vi "TermoparRef1.vi"() -> ()   [LabVIEW 2014]
uses:
  <vilib>/Analysis/baseanly.llb/Mean (DBL).vi
  <vilib>/Analysis/NI_AALBase.lvlib
panel:
  out "Forca (Kgf)":dbl format="%#_2f"
  out "Input Voltage  Cel (V)":dbl format="%#_4f"
  in  "Numeric 4":dbl step=1.0 format="%#_3f"
  in  "Numeric 3":dbl step=1.0 format="%#_2f"
  in  "Numeric 2":dbl step=0.01 format="%#_2f"
  out "Emf(Hot Thermo B - mV)":dbl
  out "Temperature B (degC)":dbl format="%#.1f"
  out "Input Voltage Thermo B (V)":dbl format="%#_4f"
  out "Emf(Thermo B - mV)":dbl
  in  "Numeric":dbl step=0.1 format="%#_3f"
  out "Emf(Hot Thermo A - mV)":dbl
  out "Temperature A (degC)":dbl format="%#.1f"
  out "Input Voltage  Thermo A (V)":dbl format="%#_4f"
  out "Emf(Thermo A - mV)":dbl
  out "LM35 temperature (degC)":dbl format="%#_3f"
  in  "stop":bool
  out "Emf(Cold - mV)":dbl
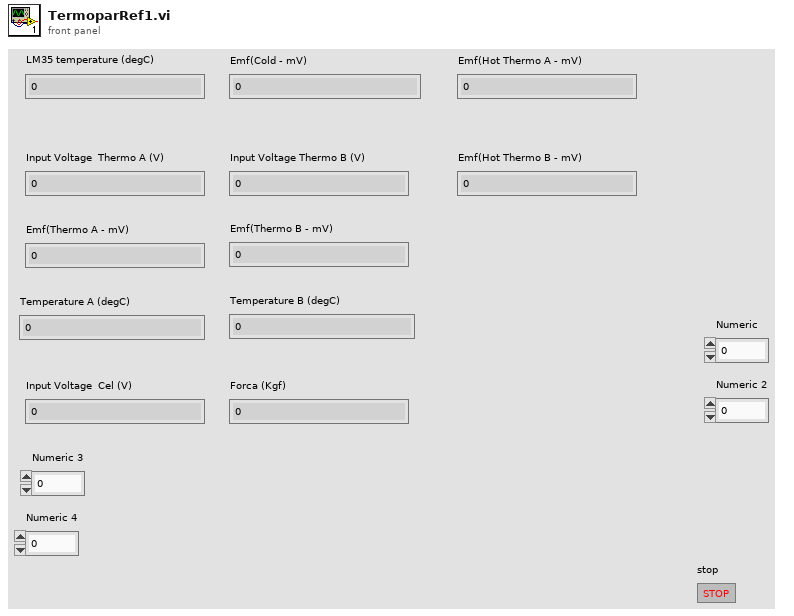
[diagram p1: front panel]
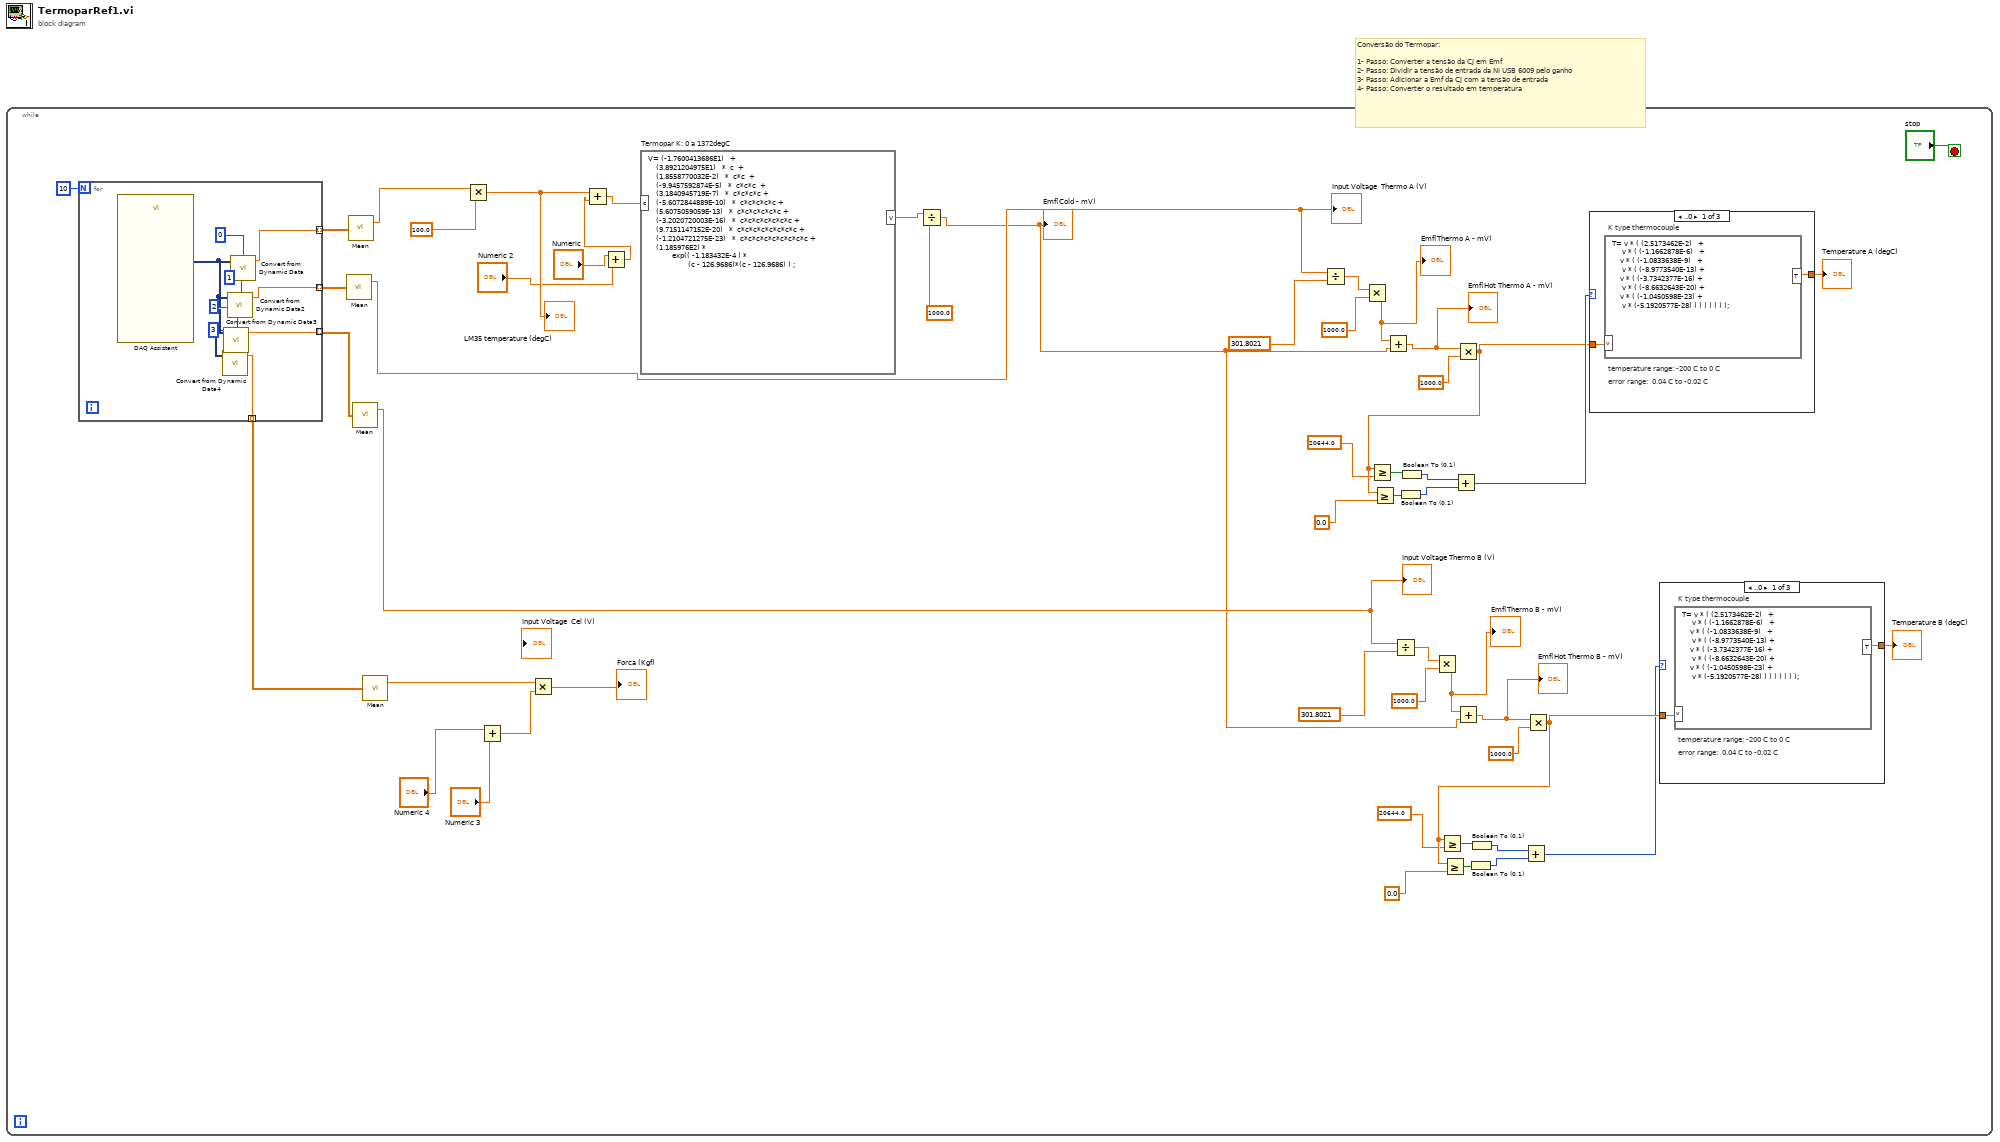
[diagram p0: block diagram]
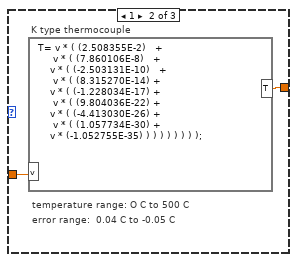
[diagram p2: hidden frame]
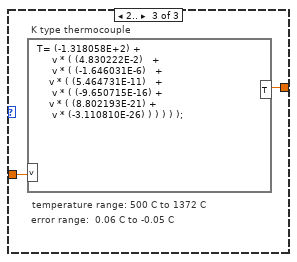
[diagram p3: hidden frame]
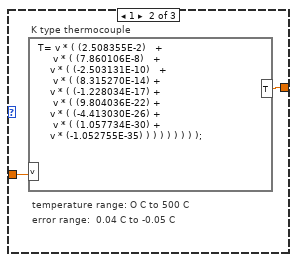
[diagram p4: hidden frame]
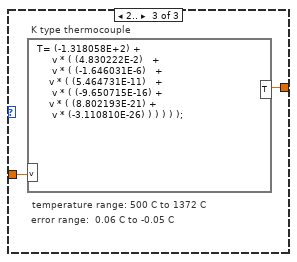
[diagram p5: hidden frame]
diagram:
  # "Conversão do Termopar:\n\n1- Passo: Converter a tensão da CJ em Emf\n2- Passo: Dividir a tensão de entrada da NI USB 6009 pelo ganho\n3- Passo: Adicionar a Emf da CJ com a tensão de entrada\n4- Passo: Converter o resultado em temperatura"
  n1 = while {
    stop <- "stop" stop-if-true
    n2 = for {
      N: 10 -> [_]
      tunnel: [w68] -> w32 mode=indexing
      tunnel: [w65] -> w31 mode=indexing
      tunnel: [w63] -> w12 mode=indexing
      tunnel: [w62] -> w2 mode=indexing
      n3 = call "DAQ Assistant"() -> ("data"=w61:dynamicdata)  [unwired: 17 in, 2 out]
      n4 = call "Convert from Dynamic Data4"("Dynamic Data Type"=w61, "Channel"=3) -> ("Scalar"=w62:dbl)  [unwired: 2 in]
      n5 = call "Convert from Dynamic Data3"("Dynamic Data Type"=w61, "Channel"=2) -> ("Scalar"=w63:dbl)  [unwired: 2 in]
      n6 = call "Convert from Dynamic Data2"("Dynamic Data Type"=w61, "Channel"=1) -> ("Scalar"=w65:dbl)  [unwired: 2 in]
      n7 = call "Convert from Dynamic Data"("Dynamic Data Type"=w61, "Channel"=0) -> ("Scalar"=w68:dbl)  [unwired: 2 in]
    }
    n8 = call-poly <vilib>:"Mean.vi"("X"=w31) -> ("mean"=w28:dbl)  [unwired: 1 out]
    "Input Voltage  Thermo A (V)" <- w28
    n9 = call-poly <vilib>:"Mean.vi"("X"=w32) -> ("mean"=w33:dbl)  [unwired: 1 out]
    n10 = call-poly <vilib>:"Mean.vi"("X"=w12) -> ("mean"=w11:dbl)  [unwired: 1 out]
    "Input Voltage Thermo B (V)" <- w11
    n11 = call-poly <vilib>:"Mean.vi"("X"=w2) -> ("mean"=w1:dbl)  [unwired: 1 out]
    n12 = Multiply(x=w33, y=100.0) -> (x*y=w30:dbl)
    "LM35 temperature (degC)" <- w30
    n13 = Add(x="Numeric 4", y="Numeric 3") -> (x+y=w6:dbl)
    n14 = Multiply(x=w1, y=w6) -> (x*y=→"Forca (Kgf)":dbl)
    n15 = Add(x="Numeric", y="Numeric 2") -> (x+y=w7:dbl)
    n16 = Add(x=w30, y=w7) -> (x+y=w29:dbl)
    n17 = formula code="V= (-1.7600413686E1)   +\n    (3.8921204975E1)   *  c  +\n    (1.8558770032E-2)   *  c*c  +\n    (-9.9457592874E-5)   *  c*c*c  +\n    (3.1840945719E-7)   *  c*c*c*c +\n    (-5.6072844889E-10)   *  c*c*c*c*c +\n    (5.6075059059E-13)   *  c*c*c*c*c*c +\n    (-3.2020720003E-16)   *  c*c*c*c*c*c*c +\n    (9.7151147152E-20)   *  c*c*c*c*c*c*c*c +\n    (-1.2104721275E-23)   *  c*c*c*c*c*c*c*c*c +\n    (1.185976E2) * \n            exp(( -1.183432E-4 ) * \n                    (c - 126.9686)*(c - 126.9686) ) ;" "Termopar K: 0 a 1372degC"("c"=w29) -> ("V"=w52:dbl)
    n18 = Divide(x=w52, y=1000.0) -> (x/y=w10:dbl)
    "Emf(Cold - mV)" <- w10
    n19 = Divide(x=w28, y=301.8021) -> (x/y=w37:dbl)
    n20 = Multiply(x=w37, y=1000.0) -> (x*y=w35:dbl)
    "Emf(Thermo A - mV)" <- w35
    n21 = Add(x=w35, y=w10) -> (x+y=w38:dbl)
    "Emf(Hot Thermo A - mV)" <- w38
    n22 = Divide(x=w11, y=301.8021) -> (x/y=w25:dbl)
    n23 = Multiply(x=w25, y=1000.0) -> (x*y=w27:dbl)
    "Emf(Thermo B - mV)" <- w27
    n24 = Multiply(x=w38, y=1000.0) -> (x*y=w39:dbl)
    n25 = Greater Or Equal?(x=w39, y=20644.0) -> (x >= y?=w46:bool)
    n26 = Greater Or Equal?(x=w39, y=0.0) -> (x >= y?=w45:bool)
    n27 = Boolean To (0,1)(Boolean=w45) -> (0, 1=w47:i16)
    n28 = Boolean To (0,1)(Boolean=w46) -> (0, 1=w48:i16)
    n29 = Add(x=w48, y=w47) -> (x+y=w42:i16)
    n30 = Add(x=w27, y=w10) -> (x+y=w24:dbl)
    "Emf(Hot Thermo B - mV)" <- w24
    n31 = Multiply(x=w24, y=1000.0) -> (x*y=w23:dbl)
    n32 = Greater Or Equal?(x=w23, y=20644.0) -> (x >= y?=w16:bool)
    n33 = Greater Or Equal?(x=w23, y=0.0) -> (x >= y?=w17:bool)
    n34 = Boolean To (0,1)(Boolean=w17) -> (0, 1=w15:i16)
    n35 = Boolean To (0,1)(Boolean=w16) -> (0, 1=w14:i16)
    n36 = Add(x=w14, y=w15) -> (x+y=w20:i16)
    n37 = case shown="..0" w42 {
      tunnel: w39 -> [w69 w71 w74]
      tunnel: [w70 w72 w73] -> w41
      frame ..0 {
        # "error range:  0.04 C to -0.02 C"
        # "temperature range: -200 C to 0 C"
        # "K type thermocouple"
        n38 = formula code="T= v * ( (2.5173462E-2)   +\n     v * ( (-1.1662878E-6)   +\n    v * ( (-1.0833638E-9)   +\n     v * ( (-8.9773540E-13) +\n    v * ( (-3.7342377E-16) +\n     v * ( (-8.6632643E-20) +\n    v * ( (-1.0450598E-23) +\n     v * (-5.1920577E-28) ) ) ) ) ) ) );"("v"=w69) -> ("T"=w70:dbl)
      }
      frame 1 {
        # "error range:  0.04 C to -0.05 C"
        # "temperature range: O C to 500 C"
        # "K type thermocouple"
        n39 = formula code="T= v * ( (2.508355E-2)   +\n     v * ( (7.860106E-8)   +\n    v * ( (-2.503131E-10)   +\n     v * ( (8.315270E-14) +\n    v * ( (-1.228034E-17) +\n     v * ( (9.804036E-22) +\n    v * ( (-4.413030E-26) +\n     v * ( (1.057734E-30) +               \n    v * (-1.052755E-35) ) ) ) ) ) ) ) );"("v"=w71) -> ("T"=w72:dbl)
      }
      frame 2.. {
        # "error range:  0.06 C to -0.05 C"
        # "temperature range: 500 C to 1372 C"
        # "K type thermocouple"
        n40 = formula code="T= (-1.318058E+2) +\n     v * ( (4.830222E-2)   +\n     v * ( (-1.646031E-6)   +\n    v * ( (5.464731E-11)   +\n     v * ( (-9.650715E-16) +\n    v * ( (8.802193E-21) +\n     v * (-3.110810E-26) ) ) ) ) );"("v"=w74) -> ("T"=w73:dbl)
      }
    }
    "Temperature A (degC)" <- w41
    n41 = case shown="..0" w20 {
      tunnel: w23 -> [w54 w56 w59]
      tunnel: [w55 w57 w58] -> w21
      frame ..0 {
        # "error range:  0.04 C to -0.02 C"
        # "temperature range: -200 C to 0 C"
        # "K type thermocouple"
        n42 = formula code="T= v * ( (2.5173462E-2)   +\n     v * ( (-1.1662878E-6)   +\n    v * ( (-1.0833638E-9)   +\n     v * ( (-8.9773540E-13) +\n    v * ( (-3.7342377E-16) +\n     v * ( (-8.6632643E-20) +\n    v * ( (-1.0450598E-23) +\n     v * (-5.1920577E-28) ) ) ) ) ) ) );"("v"=w54) -> ("T"=w55:dbl)
      }
      frame 1 {
        # "error range:  0.04 C to -0.05 C"
        # "temperature range: O C to 500 C"
        # "K type thermocouple"
        n43 = formula code="T= v * ( (2.508355E-2)   +\n     v * ( (7.860106E-8)   +\n    v * ( (-2.503131E-10)   +\n     v * ( (8.315270E-14) +\n    v * ( (-1.228034E-17) +\n     v * ( (9.804036E-22) +\n    v * ( (-4.413030E-26) +\n     v * ( (1.057734E-30) +               \n    v * (-1.052755E-35) ) ) ) ) ) ) ) );"("v"=w56) -> ("T"=w57:dbl)
      }
      frame 2.. {
        # "error range:  0.06 C to -0.05 C"
        # "temperature range: 500 C to 1372 C"
        # "K type thermocouple"
        n44 = formula code="T= (-1.318058E+2) +\n     v * ( (4.830222E-2)   +\n     v * ( (-1.646031E-6)   +\n    v * ( (5.464731E-11)   +\n     v * ( (-9.650715E-16) +\n    v * ( (8.802193E-21) +\n     v * (-3.110810E-26) ) ) ) ) );"("v"=w59) -> ("T"=w58:dbl)
      }
    }
    "Temperature B (degC)" <- w21
  }
